vi "FlatToRichtest_service_WaitResponse.vi"(5 "OutputClusterType":T1, 11 "InputCluster":T2) -> (3 "OutputCluster":T1)   [LabVIEW 2021, in "test_service_server.lvlib"]
uses:
  test_service_server.lvlib
  test_service_WaitResponse_Flat.ctl
  test_service_WaitResponse.ctl
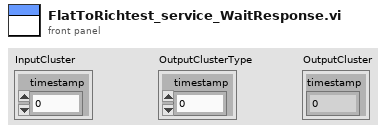
[diagram p1: front panel]
types:
  T1 = typedef "test_service_server.lvlib/test_service_WaitResponse.ctl" = cluster{"timestamp":u64}
  T2 = typedef "test_service_server.lvlib/test_service_WaitResponse_Flat.ctl" = cluster{"timestamp":u64}
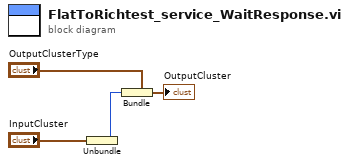
[diagram p0: block diagram]
diagram:
  n1 = Unbundle "Unbundle"("InputCluster") -> ("timestamp"=w1:u64)
  n2 = Bundle "Bundle"(cluster="OutputClusterType", "timestamp"=w1) -> (→"OutputCluster":T1)
